vi "IFw_Testbench.vi"() -> ()   [LabVIEW 2017]
uses:
  <instrlib>/_niInstr/FIFO Register Bus/v1/Host/niInstr FIFO Register Bus v1 Host.lvclass
  C:/Program Files (x86)/National Instruments/LabVIEW 2017/instr.lib/_niInstr/Instruction Framework/v1/Host/Instruction Target/niInstr Instruction Target v1 Host.lvclass
  <vilib>/FPGAPlugInAG/sbRIO-9607/niLvFpga_Open_sbRIO-9607.vi
  <vilib>/rvi/interface/common/dynamic/niFpgaDynamicAddResources.vi
  <instrlib>/_niInstr/Instruction Framework/v1/Host/Subsystem Map/Private/Lookup Single Context.vi
  <vilib>/Utility/error.llb/Error Cluster From Error Code.vi
  <vilib>/rvi/errors/niLvFpgaAdjustHostInterfaceError.vi
  <vilib>/FPGAPlugInAG/Dynamic/niLvFpga_Close_Dynamic.vi
  <vilib>/rvi/interface/nirviOpenFPGA/nirviOpenFPGA.xnode
  FPGA Bitfiles/ScaleAndLimit_FPGATarget_InstructionFrame_+7wJIgSopvQ.lvbitx
  <vilib>/rvi/interface/nirviReadWriteControl/nirviReadWriteControl.xnode
  <vilib>/rvi/interface/nirviCloseFPGA/nirviCloseFPGA.xnode
  <instrlib>/_niInstr/Instruction Framework/v1/Host/Subsystem Map/niInstr Subsystem Map v1 Host.lvclass
  <instrlib>/_niInstr/Instruction Framework/v1/Host/Instruction Target/niInstr Instruction Target v1 Host.lvclass
  NiFpgaLv.dll
  <vilib>/rvi/interface/Simulation/niFpgaSimulationCallBeginRW.vi
panel:
  out "U32":u32 format="%.0x"
  in  "SGL":sgl format="%#_13g"
  out "ScaledAI":sgl[](array[numeric])
  out "SGL":sgl
  out "error out":errorcluster
  in  "stop":bool
  in  "data":u64 format="%.0x"
  in  "address":u64
  in  "set":bool
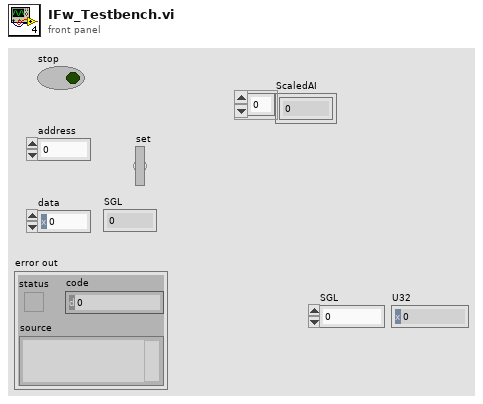
[diagram p1: front panel]
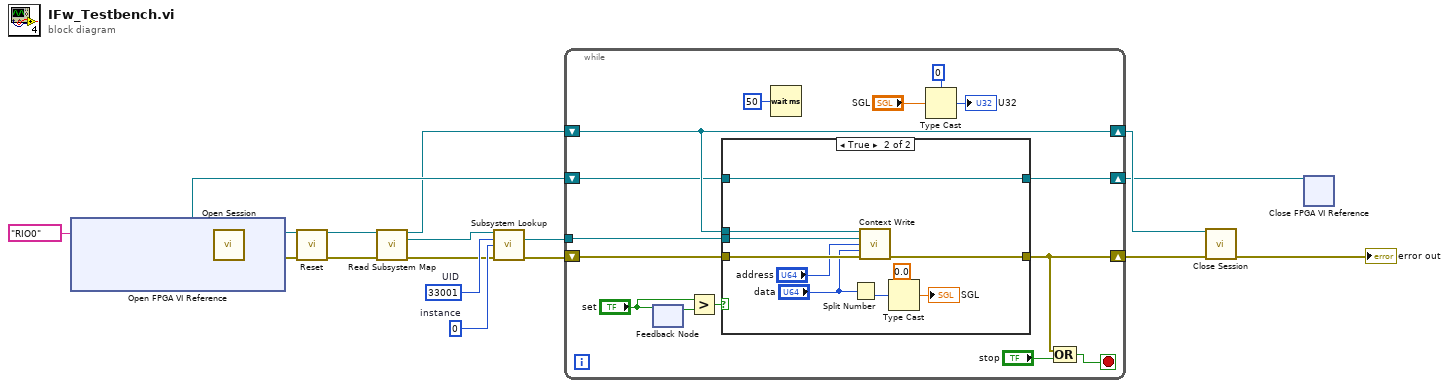
[diagram p0: block diagram]
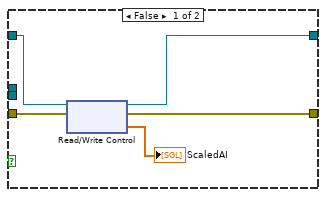
[diagram p2: hidden frame]
diagram:
  w12 = u8 0  # instance
  w13 = u16 33001  # UID
  n1 = xnode "Open FPGA VI Reference"("resource name"=tag "RIO0") -> ("FPGA VI Reference Out"=w4:refnum<k20>, "error out"=w5:errorcluster)  [unwired: 1 in]
  n2 = call <instrlib>:"Open Session.vi"("fpga ref"=w4, "error in"=w5) -> ("session out"=w8:refnum<class "niInstr FIFO Register Bus v1 Host.lvclass">, "error out"=w9:errorcluster)  [unwired: 12 in]
  n3 = call-dynamic "Reset.vi"("session in"=w8, "error in"=w9) -> ("session out"=w6:refnum<class "niInstr FIFO Register Bus v1 Host.lvclass">, "error out"=w7:errorcluster)  [unwired: 12 in]
  n4 = call <instrlib>:"Read Subsystem Map.vi"("instruction target in"=w6, "error in"=w7) -> ("instruction target out"=w3:refnum<class "niInstr FIFO Register Bus v1 Host.lvclass">, "subsystem map"=w2:refnum<class "niInstr Subsystem Map v1 Host.lvclass">, "error out"=w1:errorcluster)  [unwired: 11 in]
  n5 = call-poly <instrlib>:"Subsystem Lookup.vi"("subsystem map in"=w2, "UID"=w13, "instance"=w12, "error in"=w1) -> ("context"=w11:refnum<class "niInstr Instruction Framework Context v1 Host.lvclass">, "error out"=w10:errorcluster)  [unwired: 8 in, 2 out]
  n6 = while {
    shift-right: [w33] -> w18
    shift-left: w3 -> [w33]
    tunnel: w11 -> [w31]
    shift-right: [w24] -> w17
    shift-left: w10 -> [w32]
    shift-right: [w22] -> w14
    shift-left: w4 -> [w26]
    stop <- w23 stop-if-true
    n7 = feedback-in #1("set") -> ()
    n8 = feedback #1() -> (w30:bool)  [unwired: 1 in]
    n9 = Greater?(x="set", y=w30) -> (0:w28:bool)
    n10 = case shown="True" w28 {
      tunnel: w33 -> [_ w48]
      tunnel: w32 -> [w38 w47]
      tunnel: w31 -> [_ w46]
      tunnel: [w36 w45] -> w24
      tunnel: w26 -> [w37 w43]
      tunnel: [w35 w43] -> w22
      frame False {
        n11 = xnode "Read/Write Control"("FPGA VI Reference In"=w37, "error in"=w38) -> ("FPGA VI Reference Out"=w35:refnum<k20>, "error out"=w36:errorcluster, "ScaledAI"=→"ScaledAI":sgl[])
      }
      frame True {
        n12 = Split Number(x="data") -> (lo(x)=w41:u32)  [unwired: 1 out]
        n13 = call <instrlib>:"Context Write.vi"("instruction target in"=w48, "context in"=w46, "address"="address", "data"="data", "error in"=w47) -> ("error out"=w45:errorcluster)  [unwired: 8 in, 2 out]
        n14 = Type Cast(type=sgl 0.0, x=w41) -> (*(type *) &x=→"SGL":sgl)
      }
    }
    n15 = Wait (ms)(milliseconds to wait=u32 50) -> ()  [unwired: 1 out]
    n16 = Type Cast(type=u32 0, x="SGL") -> (*(type *) &x=→"U32":u32)
    n17 = Compound Arithmetic op=OR(w24, "stop") -> (w23:bool)
  }
  n18 = call-dynamic "Close Session.vi"("session in"=w18, "error in"=w17) -> ("error out"=→"error out":errorcluster)  [unwired: 13 in]
  n19 = xnode "Close FPGA VI Reference"("FPGA VI Reference In"=w14) -> ()  [unwired: 1 in, 1 out]
